vi "inject then hplc analysis.vi"() -> ()   [LabVIEW 2015]
uses:
  <vilib>/MakerHub/LINX/Public/Peripherals/Digital/Digital Write 1 Chan.vi
  <vilib>/MakerHub/LINX/LMH-LINX.lvlib
panel:
  in  "Arduino":refnum<visa-resource-name>="N/A"
  in  "Valve":refnum<visa-resource-name>
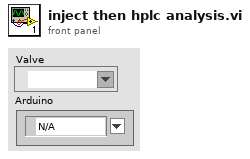
[diagram p1: front panel]
types:
  T1 = typedef "LMH-LINX.lvlib/LINX Ref.ctl" = cluster{"Platform":T2, "Interface":T3, "LINX Device Config":T4}
  T2 = typedef "LMH-LINX.lvlib/Platform.ctl" = enum16{"LINX", "myRIO"}
  T3 = typedef "LMH-LINX.lvlib/Interface.ctl" = enum16{"Serial", "TCP"}
  T4 = typedef "LMH-LINX.lvlib/Device.lvlib/LINX Device Config.ctl" = cluster{"Interface":T3, "COM Port":refnum<visa-resource-name>, "TCP Configuration":T5, "Device Family":u8, "Device ID":u8, "Device Name":string, "TCP Ref":refnum<k5>, "Channels":T6}
  T5 = typedef "LMH-LINX.lvlib/Device.lvlib/TCP Config.ctl" = cluster{"IP Address":string, "Port":u16}
  T6 = typedef "LMH-LINX.lvlib/Channels.ctl" = cluster{"DI":u8[], "DO":u8[], "AI":u8[], "AO":u8[], "PWM":u8[], "QE":u8[], "UART":u8[], "I2C 2":u8[], "SPI":u8[], "CAN":u8[], "Servo":u8[], "AI Ref (V)":dbl, "AO Ref (V)":dbl, "AO Resolution (Bits)":u8}
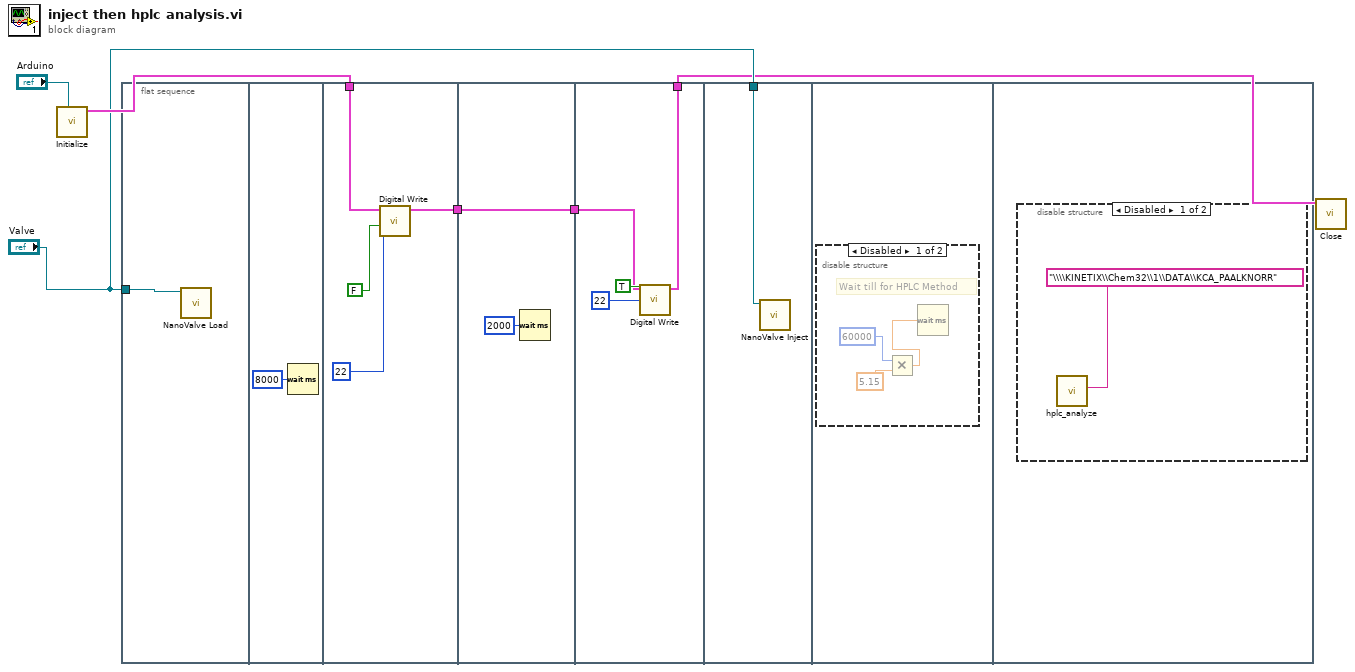
[diagram p0: block diagram]
diagram:
  n1 = call <vilib>:"Initialize.vi"("Serial Port"="Arduino") -> ("LINX Ref"=w5:T1)  [unwired: 8 in, 2 out]
  n2 = flat-sequence {
    tunnel: "Valve" -> [w7]
    tunnel: w5 -> [w10]
    tunnel: [w9] -> w2
    tunnel: [w13] -> w3
    tunnel: w2 -> [w13]
    tunnel: w3 -> [w16]
    tunnel: [w15] -> w1
    tunnel: "Valve" -> [w19]
    frame #0 {
      n3 = call "NanoValve Load.vi"("VISA resource name"=w7) -> ()  [unwired: 10 in, 1 out]
    }
    frame #1 {
      n4 = Wait (ms)(milliseconds to wait=u32 8000) -> ()  [unwired: 1 out]
    }
    frame #2 {
      n5 = call-poly <vilib>:"Digital Write.vi"("Output Value"=FALSE, "DO Channel"=u8 22, "LINX Resource"=w10) -> ("LINX Resource"=w9:T1)  [unwired: 7 in, 1 out]
    }
    frame #3 {
      n6 = Wait (ms)(milliseconds to wait=u32 2000) -> ()  [unwired: 1 out]
    }
    frame #4 {
      n7 = call-poly <vilib>:"Digital Write.vi"("Output Value"=TRUE, "DO Channel"=u8 22, "LINX Resource"=w16) -> ("LINX Resource"=w15:T1)  [unwired: 7 in, 1 out]
    }
    frame #5 {
      n8 = call "NanoValve Inject.vi"("VISA resource name"=w19) -> ()  [unwired: 10 in, 1 out]
    }
    frame #6 {
      n9 = disable-structure shown="Disabled" {
        frame Disabled {
          # "Wait till for HPLC Method"
          n10 = Multiply(x=u32 60000 ("milliseconds to wait"), y=5.15) -> (x*y=w22:dbl)
          n11 = Wait (ms)(milliseconds to wait=w22) -> ()  [unwired: 1 out]
        }
        frame Enabled {
        }
      }
    }
    frame #7 {
      n12 = disable-structure shown="Disabled" {
        frame Disabled {
          n13 = call "hplc_analyze.vi"("File Path"="\\\\KINETIX\\Chem32\\1\\DATA\\KCA_PAALKNORR") -> ()  [unwired: 11 in]
        }
        frame Enabled {
        }
      }
    }
  }
  n14 = call <vilib>:"Close.vi"("LINX Resource"=w1) -> ()  [unwired: 9 in, 2 out]
